vi "DotNETCam_CastUIEvent.vi"(11 "UIEvent":T2) -> (1 "Data":variant, 2 "ApplicationGUI out":refnum<class "DotNETCam.lvclass">, 3 "UiEventNames":T1)   [LabVIEW 2021, in "DotNETCam.lvclass"]
uses:
  DotNETCam.lvclass
  DotNETCam_UiCallBackEvents.ctl
  DotNETCam.lvclass/DotNETCam.ctl
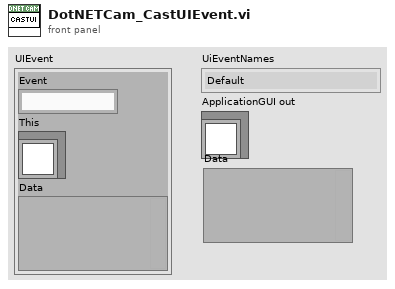
[diagram p1: front panel]
types:
  T1 = typedef "DotNETCam.lvclass/DotNETCam_UiCallBackEvents.ctl" = enum16{"Default", "PersistentDataUpdated", "Worker 1: Do Something"}
  T2 = cluster{"Event":string, "This":refnum<class>, "Data":variant}
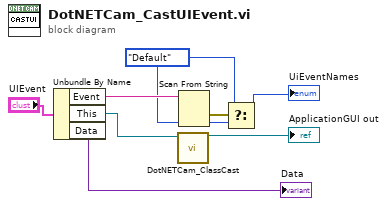
[diagram p0: block diagram]
diagram:
  w2 = DotNETCam_UiCallBackEvents."Default" ("UiEventNames")
  n1 = Unbundle By Name("UIEvent") -> ("Event"=w7:string, "This"=w6:refnum<class>, "Data"=→"Data":variant)
  n2 = call "DotNETCam_ClassCast.vi"("DotNETCam in"=w6) -> ("DotNETCam out"=→"ApplicationGUI out":refnum<class "DotNETCam.lvclass">)  [unwired: 10 in]
  n3 = Scan From String(input string=w7, default 1=w2) -> (error out=w5:errorcluster, output 1=w4:T1)  [unwired: 3 in, 2 out]
  n4 = Select(t=w2, s=w5, f=w4) -> (s? t:f=→"UiEventNames":T1)
